vi "LoopFactory.vi"(8 "error in":errorcluster, 11 "reference":refnum<vi>) -> (0 "error out":errorcluster, 3 "Loop out":refnum<class "Loop.lvclass">)   [LabVIEW 2014, in "Raspberry Pi Compatible Compiler for LabVIEW.lvlib" / "Loop.lvclass"]
uses:
  Loop.lvclass
  ForLoop/ForLoop.lvclass
  WhileLoop/WhileLoop.lvclass
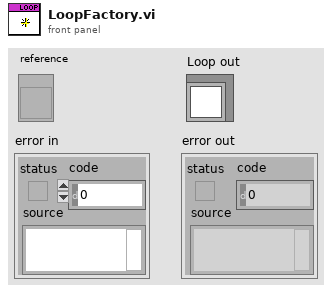
[diagram p1: front panel]
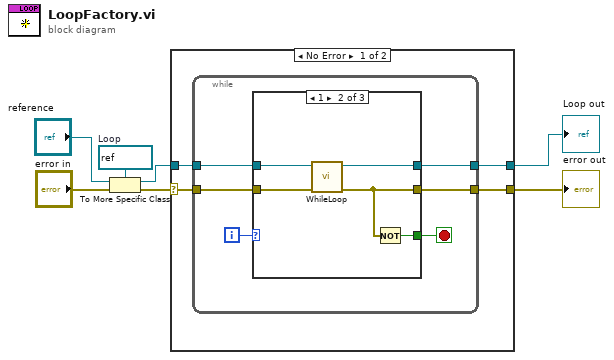
[diagram p0: block diagram]
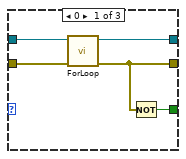
[diagram p2: hidden frame]
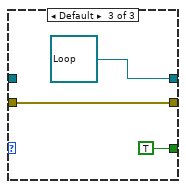
[diagram p3: hidden frame]
diagram:
  w5 = refnum<vi> refnum  # Loop
  n1 = To More Specific Class(target class=w5, reference="reference", error in="error in") -> (specific class reference=w2:refnum<vi>, error out=w3:errorcluster)
  n2 = case shown="No Error" w3 {
    selector: w3 -> [w11 w31]
    tunnel: [w9 _] -> w7
    tunnel: [w8 w31] -> w6
    tunnel: w2 -> [w10 _]
    frame No Error {
      n3 = while {
        tunnel: w11 -> [w16]
        tunnel: [w15] -> w8
        tunnel: [w14] -> w9
        tunnel: w10 -> [w12]
        i -> [w17]
        stop <- w13 stop-if-true
        n4 = case shown="1" w17 {
          tunnel: w16 -> [w19 w24 w29]
          tunnel: [w20 w25 w29] -> w15
          tunnel: [w18 w23 refnum<class "Loop.lvclass"> refnum ("Loop.lvclass")] -> w14
          tunnel: [w22 w27 TRUE] -> w13
          tunnel: w12 -> [w21 w26 _]
          frame 0 {
            n5 = call "ForLoop.vi"("error in"=w19, "reference"=w21) -> ("error out"=w20:errorcluster, "ForLoop out"=w18:refnum<class "ForLoop.lvclass">)  [unwired: 8 in]
            n6 = Not(x=w20) -> (.not. x?=w22:bool)
          }
          frame 1 {
            n7 = call "WhileLoop.vi"("error in"=w24, "reference"=w26) -> ("error out"=w25:errorcluster, "WhileLoop out"=w23:refnum<class "WhileLoop.lvclass">)  [unwired: 8 in]
            n8 = Not(x=w25) -> (.not. x?=w27:bool)
          }
          frame Default {
          }
        }
      }
    }
    frame Error {
    }
  }
  "error out" <- w6
  "Loop out" <- w7
